vi "get palettes.vi"(8 "error in (no error)":errorcluster, 11 "Refnum in":refnum<k20>) -> (0 "error out":errorcluster, 3 "palettes":T1(array[cluster]))   [LabVIEW 2020]
uses:
  <vilib>/xml/NI_XML.lvlib
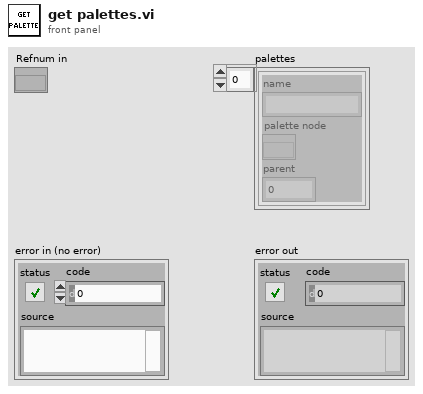
[diagram p1: front panel]
types:
  T1 = cluster{"name":string, "palette node":refnum<k20>, "parent":i32}[]
  T2 = cluster{"node text":string, "Node Reg":refnum<k20>, i32}
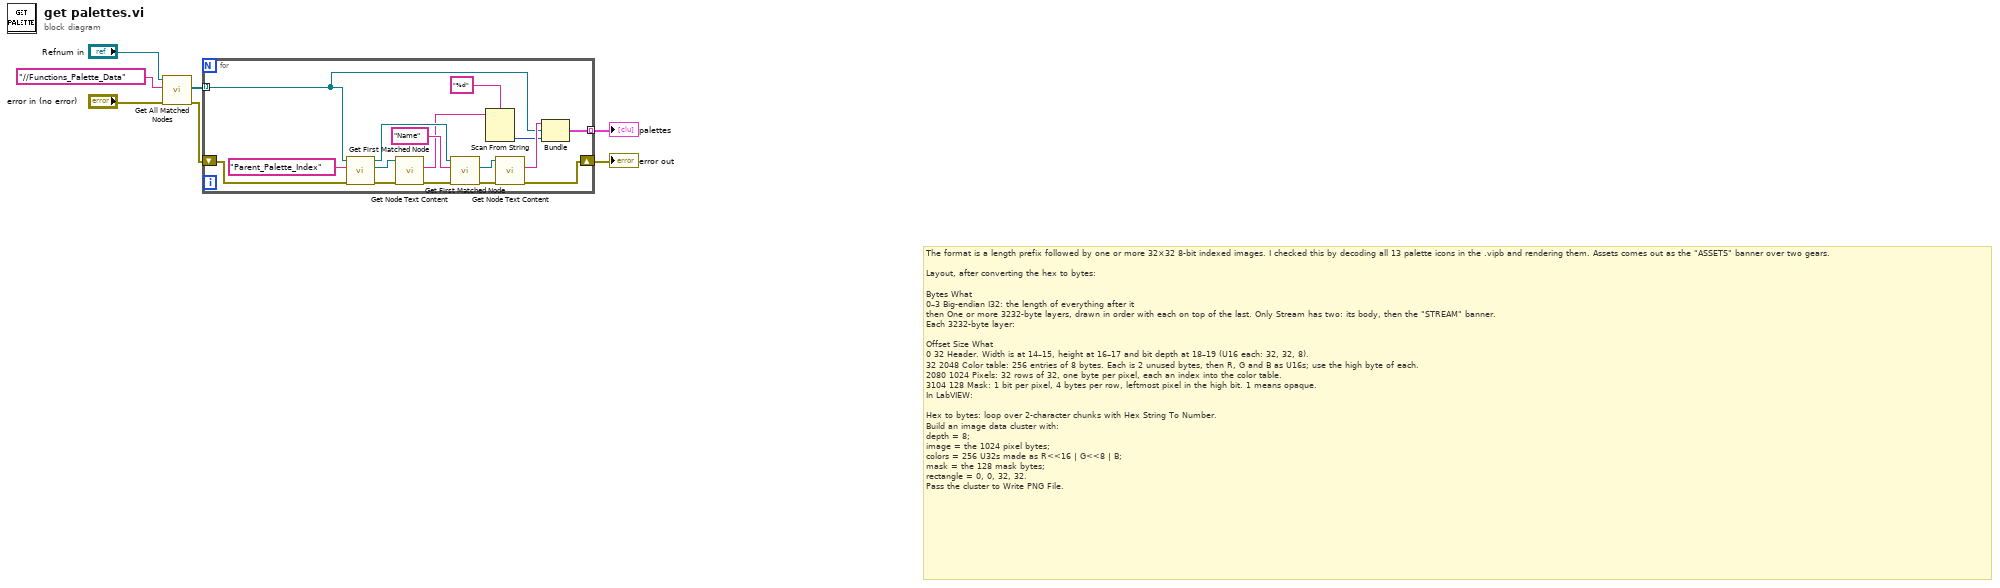
[diagram p0: block diagram]
diagram:
  # "The format is a length prefix followed by one or more 32×32 8-bit indexed images. I checked this by decoding all 13 palette icons in the .vipb and rendering them. Assets comes out as the \"ASSETS\" banner over two gears.\n\nLayout, after converting the hex to bytes:\n\nBytes\tWhat\n0–3\tBig-endian I32: the length of everything after it\nthen\tOne or more 3232-byte layers, drawn in order with each on top of the last. Only Stream has two: its body, then the \"STREAM\" banner.\nEach 3232-byte layer:\n\nOffset\tSize\tWhat\n0\t32\tHeader. Width is at 14–15, height at 16–17 and bit depth at 18–19 (U16 each: 32, 32, 8).\n32\t2048\tColor table: 256 entries of 8 bytes. Each is 2 unused bytes, then R, G and B as U16s; use the high byte of each.\n2080\t1024\tPixels: 32 rows of 32, one byte per pixel, each an index into the color table.\n3104\t128\tMask: 1 bit per pixel, 4 bytes per row, leftmost pixel in the high bit. 1 means opaque.\nIn LabVIEW:\n\nHex to bytes: loop over 2-character chunks with Hex String To Number.\nBuild an image data cluster with:\ndepth = 8;\nimage = the 1024 pixel bytes;\ncolors = 256 U32s made as R<<16 | G<<8 | B;\nmask = the 128 mask bytes;\nrectangle = 0, 0, 32, 32.\nPass the cluster to Write PNG File."
  n1 = call <vilib>:"Get All Matched Nodes.vi"("error in (no error)"="error in (no error)", "XPath expression"="//Functions_Palette_Data", "node in"="Refnum in") -> ("error out"=w4:errorcluster, "node result array"=w3:refnum<k20>[])  [unwired: 6 in, 1 out]
  n2 = for {
    tunnel: w3 -> [w8] mode=indexing
    shift-right: [w16] -> w5
    shift-left: w4 -> [w23]
    tunnel: [w10] -> w7 mode=indexing
    n3 = call <vilib>:"Get First Matched Node.vi"("error in (no error)"=w23, "XPath expression"="Parent_Palette_Index", "node in"=w8) -> ("error out"=w19:errorcluster, "node result"=w9:refnum<k20>, "node out"=w21:refnum<k20>)  [unwired: 6 in]
    n4 = call <vilib>:"Get Node Text Content.vi"("error in (no error)"=w19, "node in"=w9) -> ("error out"=w18:errorcluster, "node text"=w13:string)  [unwired: 7 in, 1 out]
    n5 = call <vilib>:"Get First Matched Node.vi"("error in (no error)"=w18, "XPath expression"="Name", "node in"=w21) -> ("error out"=w17:errorcluster, "node result"=w15:refnum<k20>)  [unwired: 6 in, 1 out]
    n6 = Scan From String(format string="%d", input string=w13) -> (output 1=w12:i32)  [unwired: 3 in, 3 out]
    n7 = call <vilib>:"Get Node Text Content.vi"("error in (no error)"=w17, "node in"=w15) -> ("error out"=w16:errorcluster, "node text"=w14:string)  [unwired: 7 in, 1 out]
    n8 = Bundle("node text"=w14, "Node Reg"=w8, w12) -> (w10:T2)  [unwired: 1 in]
  }
  "palettes" <- w7
  "error out" <- w5
